vi "Untitled 66.vi"() -> ()   [LabVIEW 2015]
uses:
  <vilib>/NXT/Dual Mode Library/Sensors/Light_On.vi
  <vilib>/NXT/Dual Mode Library/Motors/MotorOn.vi
  <vilib>/NXT/Dual Mode Library/Motors/MotorReverse.vi
  <vilib>/NXT/Dual Mode Library/Waits/Wait_Num.vi
  <vilib>/NXT/Block Support/NXT_InputPort.ctl
  <vilib>/NXT/Subs/MotorOutput.ctl
panel:
  in  "Output Port (All Ports) 7":T1=3 items=["Port A", "Port B", "Port C", "All Ports"]
  in  "Output Port (All Ports) 8":T1=3 items=["Port A", "Port B", "Port C", "All Ports"]
  in  "Output Port (All Ports) 9":T1=3 items=["Port A", "Port B", "Port C", "All Ports"]
  in  "왼쪽모터 2":T1=3 caption="Output Port" items=["Port A", "Port B", "Port C", "All Ports"]
  in  "Output Port (All Ports) 2":T1=3 items=["Port A", "Port B", "Port C", "All Ports"]
  in  "Power (75) 5":i32=75
  in  "Power (75) 3":i32=75
  in  "뒷센서":T2=2 items=["Port 1", "Port 2", "Port 3", "Port 4"]
  in  "앞센서":T2=2 items=["Port 1", "Port 2", "Port 3", "Port 4"]
  in  "stop":bool
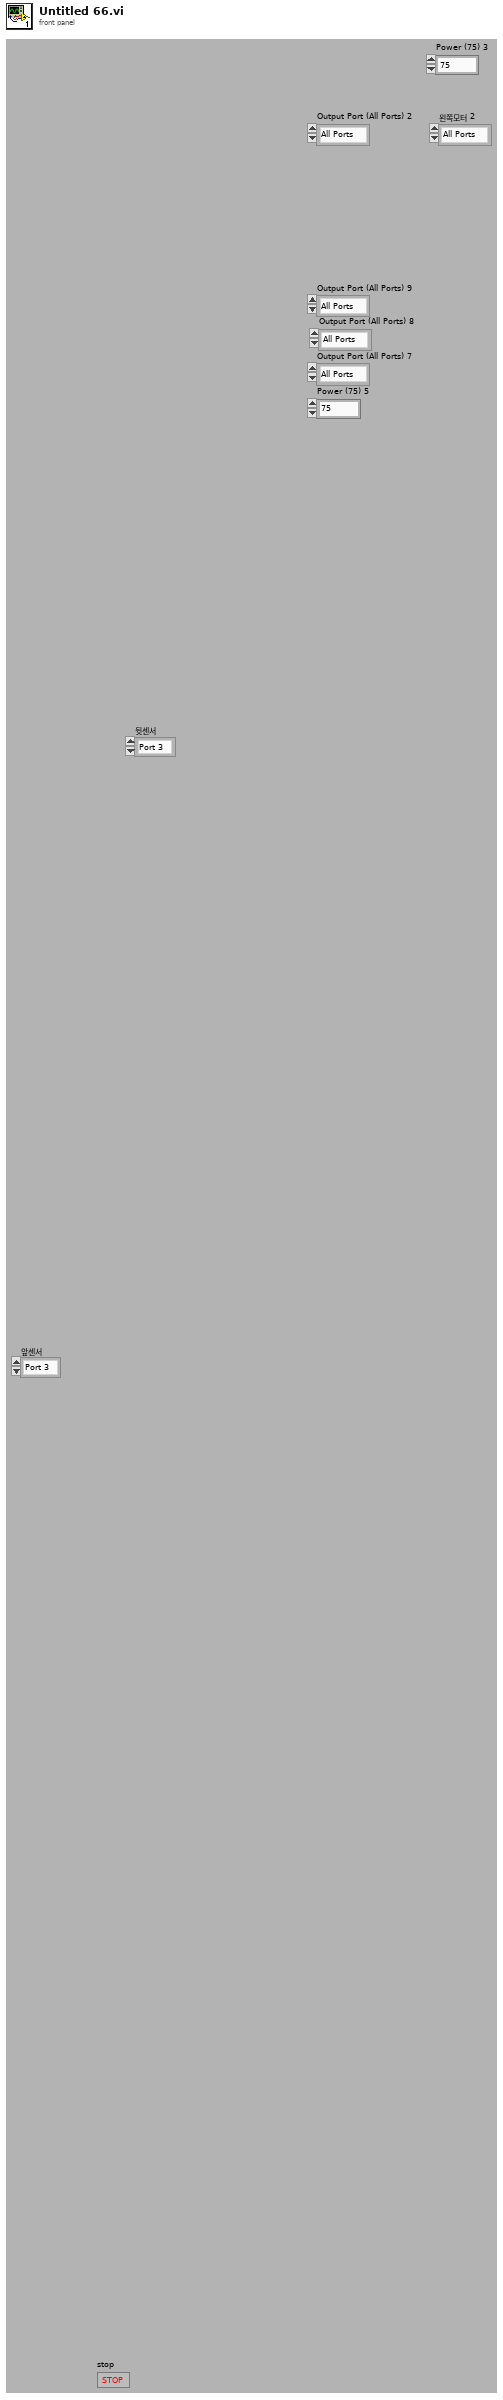
[diagram p1: front panel]
types:
  T1 = typedef "MotorOutput.ctl" = u8
  T2 = typedef "NXT_InputPort.ctl" = u8
  T3 = typedef "LVHSConnector.ctl" = cluster{"error":errorcluster, "address":string, "NXT #":i32, "Show Error":bool, "Connection":u16}
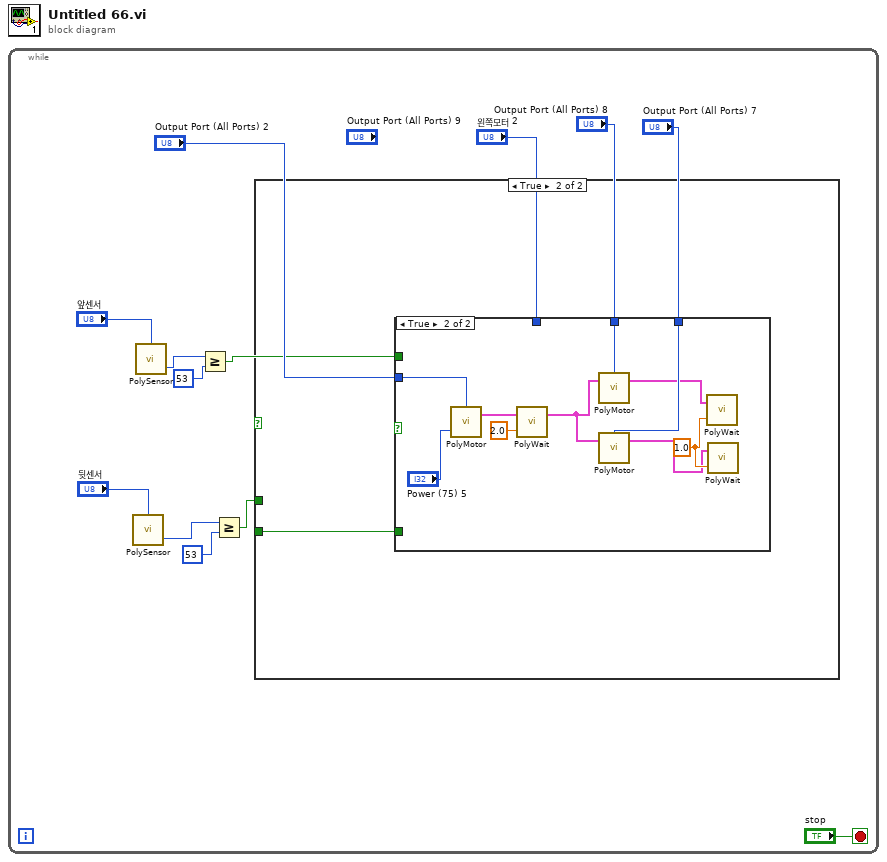
[diagram p0: block diagram]
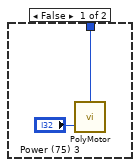
[diagram p2: hidden frame]
diagram:
  n1 = while {
    stop <- "stop" stop-if-true
    n2 = call-poly <vilib>:"PolySensor.vi"("Port (Port 3)"="뒷센서") -> ("Scaled Value"=w9:i16)  [unwired: 2 in, 1 out]
    n3 = call-poly <vilib>:"PolySensor.vi"("Port (Port 3)"="앞센서") -> ("Scaled Value"=w4:i16)  [unwired: 2 in, 1 out]
    n4 = Greater Or Equal?(x=w4, y=i16 53) -> (x >= y?=w3:bool)
    n5 = Greater Or Equal?(x=w9, y=i16 53) -> (x >= y?=w2:bool)
    n6 = case shown="True" {
      selector: _ -> [_ _]
      tunnel: w2 -> [w27 _]
      tunnel: [w27 _] -> w1
      frame False {
      }
      frame True {
      }
    }
    n7 = case shown="True" {
      selector: _ -> [_ _]
      tunnel: "Output Port (All Ports) 2" -> [_ w26]
      tunnel: "왼쪽모터 2" -> [w16 _]
      tunnel: "Output Port (All Ports) 8" -> [_ w23]
      tunnel: "Output Port (All Ports) 7" -> [_ w22]
      tunnel: w3 -> [_ _]
      tunnel: w1 -> [_ _]
      frame False {
        n8 = call-poly <vilib>:"PolyMotor.vi"("Power (75)"="Power (75) 3", "Output Port (All Ports)"=w16) -> ()  [unwired: 2 in, 1 out]
      }
      frame True {
        w18 = sgl 1.0 ("Time (sec)")
        n9 = call-poly <vilib>:"PolyMotor.vi"("Power (75)"="Power (75) 5", "Output Port (All Ports)"=w26) -> ("NXT"=w24:T3)  [unwired: 2 in]
        n10 = call-poly <vilib>:"PolyWait.vi"("Time (sec)"=sgl 2.0 ("Time (1 sec)"), "NXT"=w24) -> ("NXT"=w21:T3)  [unwired: 2 in]
        n11 = call-poly <vilib>:"PolyMotor.vi"("NXT"=w21, "Output Port (All Ports)"=w23) -> ("NXT"=w19:T3)  [unwired: 2 in]
        n12 = call-poly <vilib>:"PolyMotor.vi"("NXT"=w21, "Output Port (All Ports)"=w22) -> ("NXT"=w17:T3)  [unwired: 2 in]
        n13 = call-poly <vilib>:"PolyWait.vi"("Time (sec)"=w18, "NXT"=w19) -> ()  [unwired: 2 in, 1 out]
        n14 = call-poly <vilib>:"PolyWait.vi"("Time (sec)"=w18, "NXT"=w17) -> ()  [unwired: 2 in, 1 out]
      }
    }
  }
